vi "InitPolyTec.vi"(11 "VISA Refnum in":refnum<visa-resource-name>) -> (0 "error out":errorcluster, 2 "Success?":bool, 3 "VISA Refnum out":refnum<visa-resource-name>)   [LabVIEW 2022 SP3]
uses:
  <vilib>/Instr/_visa.llb/VISA Configure Serial Port (Instr).vi
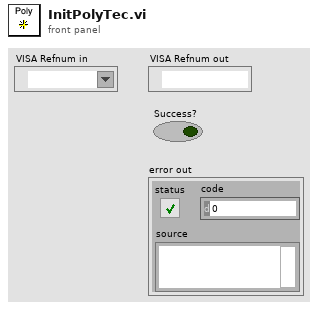
[diagram p1: front panel]
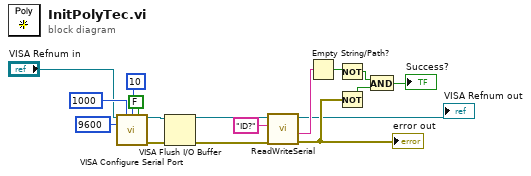
[diagram p0: block diagram]
diagram:
  n1 = call-poly "VISA Configure Serial Port"("VISA resource name"="VISA Refnum in", "timeout (10sec)"=u32 1000, "termination char\n(0xA = '\\n' = LF)"=u8 10 ("termination char\n(0xA = '\\n' = LF)"), "Enable Termination\nChar (T)"=FALSE ("Enable Termination\nChar (T)"), "baud rate (9600)"=u32 9600) -> ("VISA resource name out"=w2:refnum<visa-resource-name>, "error out"=w3:errorcluster)  [unwired: 9 in]
  n2 = VISA Flush I/O Buffer(VISA resource name=w2, error in (no error)=w3) -> (VISA resource name out=w8:refnum<visa-resource-name>, error out=w10:errorcluster)  [unwired: 1 in]
  n3 = call "ReadWriteSerial.vi"("error in (no error)"=w10, "cmd"="ID?", "VISA Refnum in"=w8) -> ("error out"=w16:errorcluster, "Reply"=w12:string, "VISA Refnum out"=→"VISA Refnum out":refnum<visa-resource-name>)  [unwired: 5 in, 1 out]
  "error out" <- w16
  n4 = Empty String/Path?(string/path=w12) -> (empty?=w13:bool)
  n5 = Not(x=w13) -> (.not. x?=w14:bool)
  n6 = Not(x=w16) -> (.not. x?=w15:bool)
  n7 = And(x=w14, y=w15) -> (x .and. y?=→"Success?":bool)
